vi "ELVIS III v1.0 RPC Reserve Resouce.vi"(5 "Owning Instrument":string, 7 "Allow multiple opens?":bool, 8 "error in (no error)":errorcluster, 9 "Session":u32, 10 "Channel Reservation List":T1, 11 "Owner":string) -> (0 "error out":errorcluster)   [LabVIEW 2021]
uses:
  <vilib>/myRIO/Common/Instrument Driver Framework/ELVIS III v1.0/Resource Manager/typedefs/ELVIS III v1.0 Channel Reservation List.ctl
  <vilib>/myRIO/Common/Instrument Driver Framework/ELVIS III v1.0/Resource Manager/typedefs/ELVIS III v1.0 Channel Reservation Info.ctl
  <vilib>/myRIO/Common/Instrument Driver Framework/ELVIS III v1.0/Resource Manager/typedefs/ELVIS III v1.0 Connector List.ctl
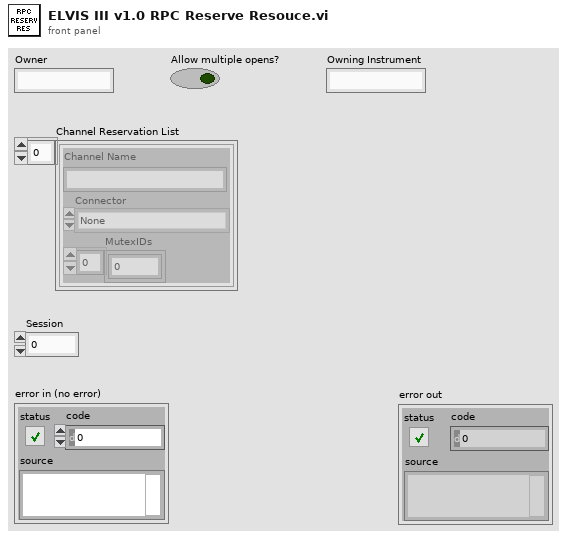
[diagram p1: front panel]
types:
  T1 = typedef "ELVIS III v1.0 Channel Reservation List.ctl" = T2[]
  T2 = typedef "ELVIS III v1.0 Channel Reservation Info.ctl" = cluster{"Channel Name":string, "Connector":T3, "MutexIDs":u32[]}
  T3 = typedef "ELVIS III v1.0 Connector List.ctl" = enum32{"None", "ConnectorA", "ConnectorB"}
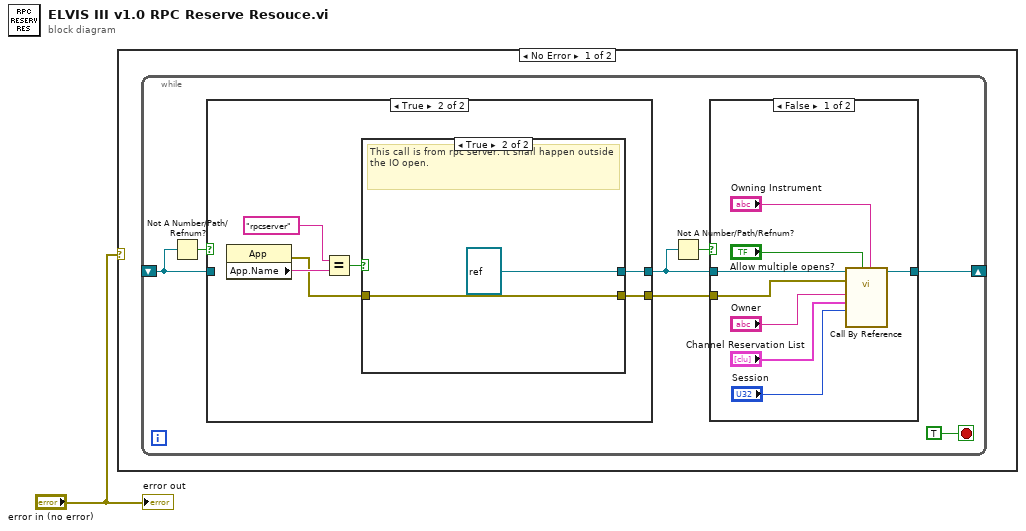
[diagram p0: block diagram]
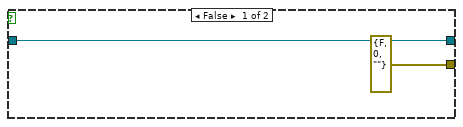
[diagram p2: hidden frame]
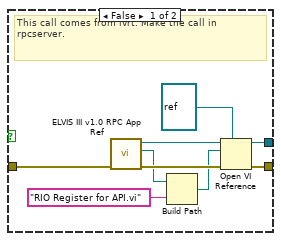
[diagram p3: hidden frame]
diagram:
  n1 = case shown="No Error" "error in (no error)" {
    frame No Error {
      n2 = while {
        shift-right: [w5] -> _
        shift-left: _ -> [w3]
        stop <- TRUE stop-if-true
        n3 = Not A Number/Path/Refnum?(number/path/refnum=w3) -> (NaN/Path/Refnum?=w4:bool)
        n4 = case shown="True" w4 {
          tunnel: [w10 w13] -> w7
          tunnel: w3 -> [w10 _]
          tunnel: [errorcluster {"status"=FALSE, "code"=0, "source"=""} ("error out") w11] -> w2
          frame False {
          }
          frame True {
            n5 = property class="App"() -> (error out=w12:errorcluster, "App.Name"=w16:string)  [unwired: 2 in, 1 out]
            n6 = Equal?(x="rpcserver" ("Application:Name"), y=w16) -> (x = y?=w15:bool)
            n7 = case shown="True" w15 {
              tunnel: [w23 refnum<vi> refnum ("type specifier VI Refnum (for type only)")] -> w13
              tunnel: w12 -> [w21 w26]
              tunnel: [w22 w26] -> w11
              frame False {
                # "This call comes from lvrt. Make the call in rpcserver."
                n8 = call <vilib>:"ELVIS III v1.0 RPC App Ref.vi"() -> ("Lib Path"=w20:path, "RPC Reference"=w18:refnum<vi>)  [unwired: 10 in]
                n9 = Build Path(base path=w20, name or relative path="RIO Register for API.vi") -> (appended path=w17:path)
                n10 = Open VI Reference(type specifier VI Refnum (for type only)=refnum<vi> refnum, application reference (local)=w18, vi path=w17, error in (no error)=w21) -> (vi reference=w23:refnum<vi>, error out=w22:errorcluster)  [unwired: 2 in]
              }
              frame True {
                # "This call is from rpc server. It shall happen outside the IO open."
              }
            }
          }
        }
        n11 = Not A Number/Path/Refnum?(number/path/refnum=w7) -> (NaN/Path/Refnum?=w8:bool)
        n12 = case shown="False" w8 {
          tunnel: w7 -> [w34 w35]
          tunnel: [w33 w35] -> w5
          tunnel: w2 -> [w32 _]
          frame False {
            n13 = call-by-ref "?"(reference=w34, error in=w32, "Owning Instrument"="Owning Instrument", "Allow multiple opens?"="Allow multiple opens?", "Session"="Session", "Channel Reservation List"="Channel Reservation List", "Owner"="Owner") -> (reference out=w33:refnum<vi>)  [unwired: 6 in, 2 out]
          }
          frame True {
            # "The call is not available. The target is installed by 19.0. Ignore for backward compatibility."
          }
        }
      }
    }
    frame Error {
    }
  }
  "error out" <- "error in (no error)"
